vi "Read_DI_Not.vi"(8 "error in (no error)":errorcluster caption="错误输入（无错误）", 11 "Name":string[](array[string])) -> (0 "DI":bool[](array[boolean]), 3 "error":bool)   [LabVIEW 2017]
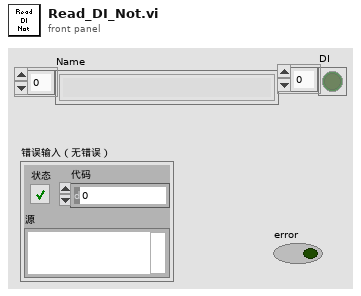
[diagram p1: front panel]
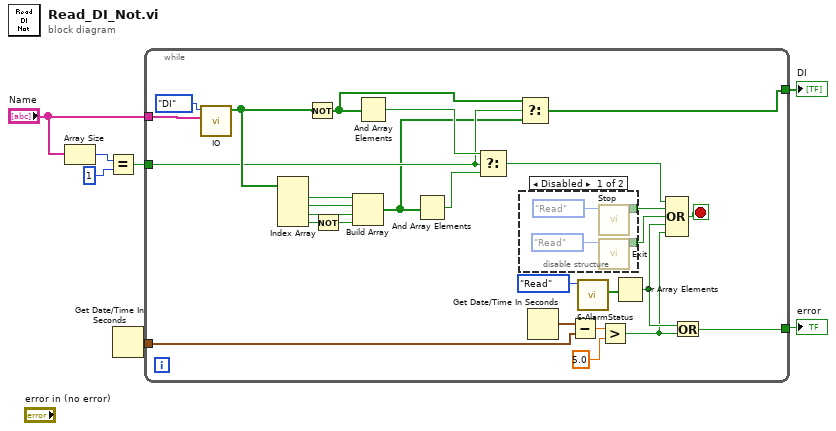
[diagram p0: block diagram]
diagram:
  n1 = Array Size(array="Name") -> (size(s)=w3:i32)
  n2 = Equal?(x=w3, y=1) -> (x = y?=w1:bool)
  n3 = Get Date/Time In Seconds() -> (seconds since 1Jan1904=w6:timestamp)
  n4 = while {
    tunnel: "Name" -> [w30]
    tunnel: w6 -> [w27]
    tunnel: [w23] -> w7
    tunnel: [w10] -> w5
    tunnel: w1 -> [w11]
    stop <- w31 stop-if-true
    n5 = call "IO.vi"("IO Name"=w30, "IO?"=enum16{"DI", "DO"}."DI") -> ("DI"=w13:bool[])  [unwired: 7 in, 2 out]
    n6 = Index Array(array=w13) -> (element #1=w15:bool, element #2=w16:bool, element #3=w17:bool, element #4=w18:bool)  [unwired: 4 in]
    n7 = Not(x=w13) -> (.not. x?=w9:bool[])
    n8 = Not(x=w18) -> (.not. x?=w19:bool)
    n9 = Build Array(w15, w16, w17, w19) -> (w8:bool[])
    n10 = And Array Elements(Boolean array=w9) -> (logical AND=w12:bool)
    n11 = And Array Elements(Boolean array=w8) -> (logical AND=w14:bool)
    n12 = Select(t=w12, s=w11, f=w14) -> (s? t:f=w20:bool)
    n13 = Select(t=w9, s=w11, f=w8) -> (s? t:f=w10:bool[])
    n14 = disable-structure shown="Disabled" {
      disable-tunnel: [w36 _] -> w33
      disable-tunnel: [w35 _] -> w32
      frame Disabled {
        n15 = call "Stop.vi"("Step"=enum16{"Initial", "Write", "Read"}."Read") -> ("Stop Out"=w35:bool)  [unwired: 9 in, 1 out]
        n16 = call "Exit.vi"("Step"=enum16{"Initial", "Write", "Read"}."Read" ("step")) -> ("Exit Out"=w36:bool)  [unwired: 9 in, 1 out]
      }
      frame Enabled {
      }
    }
    n17 = Get Date/Time In Seconds() -> (seconds since 1Jan1904=w28:timestamp)
    n18 = Subtract(x=w28, y=w27) -> (x-y=w29:dbl)
    n19 = call "6-AlarmStatus.vi"("Step"=enum16{"Initial", "Write", "Read"}."Read") -> ("AlarmValue Out"=w24:bool[])  [unwired: 9 in, 1 out]
    n20 = Greater?(x=w29, y=5.0) -> (0:w21:bool)
    n21 = Or Array Elements(Boolean array=w24) -> (logical OR=w22:bool)
    n22 = Compound Arithmetic op=OR ("复合运算")(w20, w32, w33, w22, w21) -> (w31:bool)
    n23 = Or(x=w22, y=w21) -> (x .or. y?=w23:bool)
  }
  "error" <- w7
  "DI" <- w5
